vi "Center Image Calibrate.vi"(3 "error in":errorcluster, 5 "Image In":T1) -> (0 "error out":errorcluster, 1 "Objects Array":cluster{"X Coord":dbl[], "Y Coord":dbl[]}[](array[cluster]), 2 "Image Out (duplicate)":T1)   [LabVIEW 2009]
uses:
  <vilib>/vision/Image Controls.llb/IMAQ Image.ctl
  <vilib>/vision/NI_Vision_Development_Module.lvlib
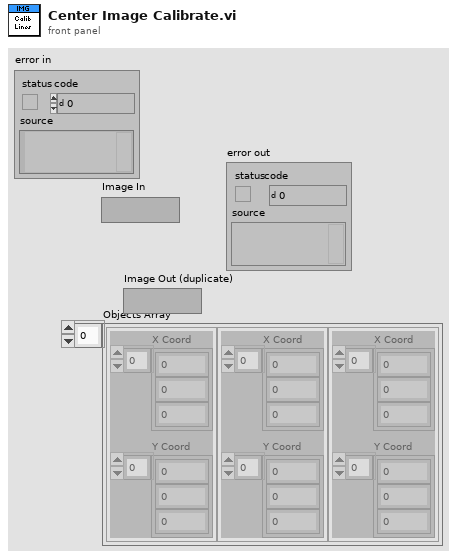
[diagram p1: front panel]
types:
  T1 = typedef "IMAQ Image.ctl" = refnum<image>
  T2 = enum32{"AutoM", "Close", "Dilate", "Erode", "Gradient", "Gradient out", "Gradient in", "Hit miss", "Open", "PClose", "POpen", "Thick", "Thin"}
  T3 = cluster{"Measurement Parameter":i32, "Range Lower Value":dbl, "Range Upper Value":dbl, "Range":bool, "Measurement Type":bool}[]
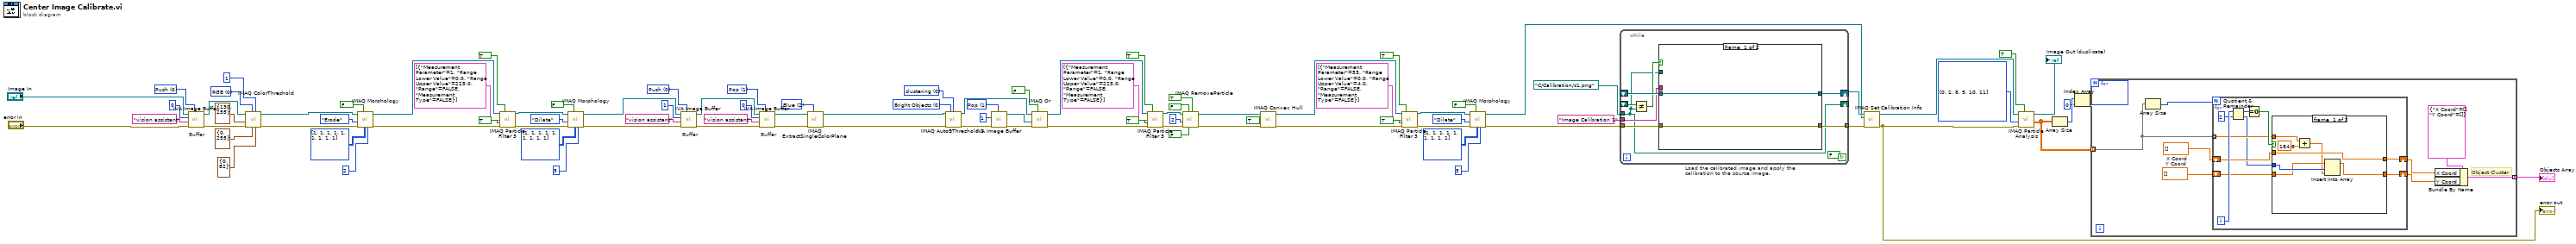
[diagram p0: block diagram]
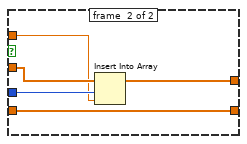
[diagram p2: hidden frame]
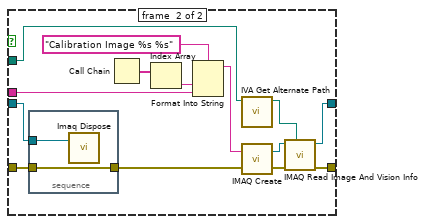
[diagram p3: hidden frame]
diagram:
  w13 = i32[] [0, 1, 8, 9, 10, 11] items=["Center of Mass X", "Center of Mass Y", "First Pixel X", "First Pixel Y", "Bounding Rect Left", "Bounding Rect Top", "Bounding Rect Right", "Bounding Rect Bottom", "Max Feret Diameter Start X", "Max Feret Diameter Start Y", "Max Feret Diameter End X", "Max Feret Diameter End Y", "Max Horiz. Segment Length Left", "Max Horiz. Segment Length Right", "Max Horiz. Segment Length Row", "-", "Bounding Rect Width", "Bounding Rect Height", "Bounding Rect Diagonal", "Perimeter", "Convex Hull Perimeter", "Holes' Perimeter", "Max Feret Diameter", "Equivalent Ellipse Major Axis", "Equivalent Ellipse Minor Axis", "Equivalent Ellipse Minor Axis (Feret)", "Equivalent Rect Long Side", "Equivalent Rect Short Side", "Equivalent Rect Diagonal", "Equivalent Rect Short Side (Feret)", "Average Horiz. Segment Length", "Average Vert. Segment Length", "Hydraulic Radius", "Waddel Disk Diameter", "-", "Area", "Holes' Area", "Particle & Holes' Area", "Convex Hull Area", "Image Area", "-", "Number of Holes", "Number of Horiz. Segments", "Number of Vert. Segments", "-", "Orientation", "Max Feret Diameter Orientation", "-", "% Area/Image Area", "% Area/(Particle & Holes' Area)", "Ratio of Equivalent Ellipse Axes", "Ratio of Equivalent Rect Sides", "-", "Elongation Factor", "Compactness Factor", "Heywood Circularity Factor", "Type Factor", "-", "Sum X", "Sum Y", "Sum XX", "Sum XY", "Sum YY", "Sum XXX", "Sum XXY", "Sum XYY", "Sum YYY", "-", "Moment of Inertia XX", "Moment of Inertia XY", "Moment of Inertia YY", "Moment of Inertia XXX", "Moment of Inertia XXY", "Moment of Inertia XYY", "Moment of Inertia YYY", "Norm. Moment of Inertia XX", "Norm. Moment of Inertia XY", "Norm. Moment of Inertia YY", "Norm. Moment of Inertia XXX", "Norm. Moment of Inertia XXY", "Norm. Moment of Inertia XYY", "Norm. Moment of Inertia YYY", "Hu Moment 1", "Hu Moment 2", "Hu Moment 3", "Hu Moment 4", "Hu Moment 5", "Hu Moment 6", "Hu Moment 7"] ("Real-World Measurements")
  w48 = u16 1 items=["Push", "Pop", "Reset"] ("Function")
  w50 = 0 items=["clustering", "entropy", "metric", "moments", "inter-class variance"] ("Method")
  w51 = u32 0 items=["Bright Objects", "Dark Objects"] ("Look For")
  w56 = 2 items=["Red", "Green", "Blue", "Hue", "Saturation", "Luminance", "Value", "Intensity"] ("Color Plane")
  w59 = u16 1 items=["Push", "Pop", "Reset"] ("Function")
  w64 = u16 0 items=["Push", "Pop", "Reset"] ("Function")
  w89 = u16 0 items=["RGB", "HSL", "HSV", "HSI"] ("Color Mode")
  w93 = u16 0 items=["Push", "Pop", "Reset"] ("Function")
  # "Buffer"
  # "Buffer"
  # "Buffer"
  n1 = call <vilib>:"IVA Image Buffer.vi"("Function"=w93, "error in (no error)"="error in", "Prefix"="vision assistant", "Buffer #"=0, "Image In"="Image In") -> ("error out"=w94:errorcluster, "Image Out"=w85:T1)  [unwired: 5 out]
  n2 = call "IMAQ ColorThreshold"("Blue or Luma or Val or Inten Range"=cluster{"Lower value":i32, "Upper value":i32} {"Lower value"=0, "Upper value"=82}, "Replace Value"=1, "Green or Sat Range"=cluster{"Lower value":i32, "Upper value":i32} {"Lower value"=0, "Upper value"=255}, "Color Mode"=w89, "error in (no error)"=w94, "Red or Hue Range"=cluster{"Lower value":i32, "Upper value":i32} {"Lower value"=130, "Upper value"=255}, "Image Src"=w85) -> ("error out"=w84:errorcluster, "Image Dst Out"=w79:T1)  [unwired: 1 in, 2 out]
  n3 = call "IMAQ Morphology"("Number of iterations (1)"=2, "Structuring Element"=i32[][] [[1, 1, 1], [1, 1, 1], [1, 1, 1]], "Square/Hexa (Square)"=FALSE, "error in (no error)"=w84, "Operation"=T2."Erode", "Image Src"=w79) -> ("error out"=w78:errorcluster, "Image Dst Out"=w74:T1)  [unwired: 1 in, 3 out]
  n4 = call "IMAQ Particle Filter 3"("Image Src"=w74, "Connectivity 4/8 (8)"=TRUE, "Selection Values"=T3 [{"Measurement Parameter"=1, "Range Lower Value"=0.0, "Range Upper Value"=225.0, "Range"=FALSE, "Measurement Type"=FALSE}], "Keep/Remove Particles (F)"=TRUE ("Keep/Remove Particles"), "error in (no error)"=w78) -> ("Image Dst Out"=w68:T1, "error out"=w75:errorcluster)  [unwired: 4 in, 5 out]
  n5 = call "IMAQ Morphology"("Number of iterations (1)"=5, "Structuring Element"=i32[][] [[1, 1, 1], [1, 1, 1], [1, 1, 1]], "Square/Hexa (Square)"=FALSE, "error in (no error)"=w75, "Operation"=T2."Dilate", "Image Src"=w68) -> ("error out"=w67:errorcluster, "Image Dst Out"=w66:T1)  [unwired: 1 in, 3 out]
  n6 = call <vilib>:"IVA Image Buffer.vi"("Function"=w64, "error in (no error)"=w67, "Prefix"="vision assistant", "Buffer #"=1, "Image In"=w66) -> ("error out"=w65:errorcluster, "Image Out"=w61:T1)  [unwired: 5 out]
  n7 = call <vilib>:"IVA Image Buffer.vi"("Function"=w59, "error in (no error)"=w65, "Prefix"="vision assistant", "Buffer #"=0, "Image In"=w61) -> ("error out"=w60:errorcluster, "Image Out"=w55:T1)  [unwired: 5 out]
  n8 = call "IMAQ ExtractSingleColorPlane"("Color Plane"=w56, "error in (no error)"=w60, "Image Src"=w55) -> ("error out"=w54:errorcluster, "Image Dst Out"=w53:T1)  [unwired: 1 in, 6 out]
  n9 = call "IMAQ AutoBThreshold 2"("Image Src"=w53, "Look For (Bright Objects)"=w51, "Method (clustering)"=w50, "error in (no error)"=w54) -> ("Image Dst Out"=w44:T1, "error out"=w52:errorcluster)  [unwired: 4 in, 6 out]
  n10 = call <vilib>:"IVA Image Buffer.vi"("Function"=w48, "error in (no error)"=w52, "Buffer #"=1) -> ("error out"=w45:errorcluster, "Image Out"=w46:T1)  [unwired: 2 in, 5 out]
  n11 = call "IMAQ Or"("Or/Nor (Or)"=FALSE, "error in (no error)"=w45, "Image Src B"=w46, "Image Src A"=w44) -> ("error out"=w43:errorcluster, "Image Dst Out"=w39:T1)  [unwired: 2 in, 4 out]
  n12 = call "IMAQ Particle Filter 3"("Image Src"=w39, "Connectivity 4/8 (8)"=TRUE, "Selection Values"=T3 [{"Measurement Parameter"=1, "Range Lower Value"=0.0, "Range Upper Value"=225.0, "Range"=FALSE, "Measurement Type"=FALSE}], "Keep/Remove Particles (F)"=TRUE ("Keep/Remove Particles"), "error in (no error)"=w43) -> ("Image Dst Out"=w33:T1, "error out"=w40:errorcluster)  [unwired: 4 in, 5 out]
  n13 = call "IMAQ RemoveParticle"("Connectivity 4/8 (8)"=TRUE, "Low Pass/High Pass (Low)"=FALSE, "Square/Hexa (Square)"=FALSE, "error in (no error)"=w40, "Number of Erosion"=2, "Image Src"=w33) -> ("error out"=w32:errorcluster, "Image Dst Out"=w31:T1)  [unwired: 1 in, 3 out]
  n14 = call "IMAQ Convex Hull"("error in (no error)"=w32, "Connectivity 4/8 (8)"=TRUE, "Image Src"=w31) -> ("error out"=w29:errorcluster, "Image Dst Out"=w25:T1)  [unwired: 1 in, 6 out]
  n15 = call "IMAQ Particle Filter 3"("Image Src"=w25, "Connectivity 4/8 (8)"=TRUE, "Selection Values"=T3 [{"Measurement Parameter"=53, "Range Lower Value"=0.0, "Range Upper Value"=4.0, "Range"=FALSE, "Measurement Type"=FALSE}], "Keep/Remove Particles (F)"=TRUE ("Keep/Remove Particles"), "error in (no error)"=w29) -> ("Image Dst Out"=w19:T1, "error out"=w26:errorcluster)  [unwired: 4 in, 5 out]
  n16 = call "IMAQ Morphology"("Number of iterations (1)"=5, "Structuring Element"=i32[][] [[1, 1, 1], [1, 1, 1], [1, 1, 1]], "Square/Hexa (Square)"=FALSE, "error in (no error)"=w26, "Operation"=T2."Dilate", "Image Src"=w19) -> ("error out"=w18:errorcluster, "Image Dst Out"=w15:T1)  [unwired: 1 in, 3 out]
  n17 = while "Load the calibrated image and apply the calibration to the source image." {
    shift-right: [w103] -> w17
    shift-left: _ -> [w102]
    tunnel: [w100] -> w16
    tunnel: w18 -> [w99]
    tunnel: path "C:/Calibration/c1.png" ("File Path") -> [w95]
    tunnel: "Image Calibration 1" ("Step Name") -> [w98]
    shift-right: [w95] -> _
    shift-left: _ -> [w97]
    stop <- FALSE continue-if-true
    n18 = Not Equal?(x=w97, y=w95) -> (x != y?=w96:bool)
    n19 = case shown="True" w96 {
      tunnel: [w105 w117] -> w103
      tunnel: w102 -> [w105 w109]
      tunnel: [w104 w114] -> w100
      tunnel: w99 -> [w104 w110]
      tunnel: w95 -> [_ w107]
      tunnel: w98 -> [_ w111]
      frame #0 {
      }
      frame #1 {
        n20 = stacked-sequence {
          tunnel: w110 -> [w120]
          tunnel: w109 -> [w121]
          tunnel: [w120] -> w108
          frame #0 {
            n21 = call "Imaq Dispose"("Image"=w121) -> ()  [unwired: 2 in, 4 out]
          }
        }
        n22 = Call Chain() -> (call chain=w113:string[])
        n23 = Index Array(array=w113) -> (element=w112:string)  [unwired: 1 in]
        n24 = Format Into String(format string="Calibration Image %s %s" ("Image Name"), w112, w111) -> (resulting string=w119:string)  [unwired: 2 in, 1 out]
        n25 = call <vilib>:"IVA Get Alternate Path.vi"("Path In"=w107) -> ("Path Out"=w106:path)  [unwired: 10 out]
        n26 = call "IMAQ Create"("Image Name"=w119, "error in (no error)"=w108) -> ("New Image"=w116:T1, "error out"=w115:errorcluster)  [unwired: 2 in, 1 out]
        n27 = call "IMAQ Read Image And Vision Info"("File Path"=w106, "error in (no error)"=w115, "Image"=w116) -> ("error out"=w114:errorcluster, "Image Out"=w117:T1)  [unwired: 1 in, 6 out]
      }
    }
  }
  n28 = call "IMAQ Set Calibration Info"("error in (no error)"=w16, "Image Dst"=w15, "Image Src"=w17) -> ("error out"=w5:errorcluster, "Calibrated Image"=w12:T1)  [unwired: 1 in, 6 out]
  "error out" <- w5
  n29 = call "IMAQ Particle Analysis"("Connectivity 4/8 (8)"=TRUE, "error in (no error)"=w5, "Real-World Measurements"=w13, "Image"=w12) -> ("Particle Measurements (Real-World)"=w7:dbl[][], "Image Out (duplicate)"=→"Image Out (duplicate)":T1)  [unwired: 1 in, 5 out]
  n30 = Array Size(array=w7) -> (size(s)=w10:i32[])
  n31 = Index Array(array=w10, index=0) -> (element=w8:i32)
  n32 = for {
    N: w8 -> [_]
    tunnel: w7 -> [w126] mode=indexing
    tunnel: [w122] -> w6 mode=indexing
    w127 = dbl[] []  # Y Coord
    w128 = dbl[] []  # X Coord
    # "Object Cluster"
    n33 = Array Size(array=w126) -> (size(s)=w129:i32)
    n34 = for {
      N: w129 -> [_]
      tunnel: w126 -> [w133] mode=indexing
      shift-right: [w131] -> w124
      shift-left: w128 -> [w135]
      shift-right: [w130] -> w123
      shift-left: w127 -> [w134]
      i -> [w139]
      n35 = Quotient & Remainder(x=w139, y=2) -> (x-y*floor(x/y)=w137:i32, floor(x/y)=w132:i32)
      n36 = Equal To 0?(x=w137) -> (x = 0?=w136:bool)
      n37 = case shown="False" w136 {
        tunnel: w135 -> [w145 w151]
        tunnel: w134 -> [w144 w147]
        tunnel: w133 -> [w141 w148]
        tunnel: w132 -> [w146 w150]
        tunnel: [w145 w149] -> w131
        tunnel: [w143 w147] -> w130
        frame #0 {
          n38 = Add(x=w141, y=184.0) -> (x+y=w140:dbl)
          n39 = Insert Into Array(array=w144, index=w146, new element=w140) -> (w143:dbl[])
        }
        frame #1 {
          n40 = Insert Into Array(array=w151, index=w150, new element=w148) -> (w149:dbl[])
        }
      }
    }
    n41 = Bundle By Name(cluster=cluster{"X Coord":dbl[], "Y Coord":dbl[]} {"X Coord"=[], "Y Coord"=[]}, "X Coord"=w124, "Y Coord"=w123) -> (w122:cluster{"X Coord":dbl[], "Y Coord":dbl[]})
  }
  "Objects Array" <- w6
